vi "8_2.vi"() -> ()   [LabVIEW 2022 SP3]
panel:
  in  "Text.Font:Bold":bool
  in  "Text.Text Colors:Text Color":u32(colorbox)
  out "Text.Selection:Start":u32
  out "Text.Selection:End":u32
  in  "font size":dbl=17.0
  in  "stop":bool
  in  "String":string="Lorem ipsum dolor sit amet, consectetur adipiscing elit, sed do eiusmod tempor incididunt ut labore et dolore magna aliqua. Ut enim ad minim veniam, quis nostrud exercitation ullamco laboris nisi ut aliquip ex ea commodo consequat. Duis aute irure dolor in reprehenderit in voluptate velit esse cillum dolore eu fugiat nulla pariatur. Excepteur sint occaecat cupidatat non proident, sunt in culpa qui officia deserunt mollit anim id est laborum."
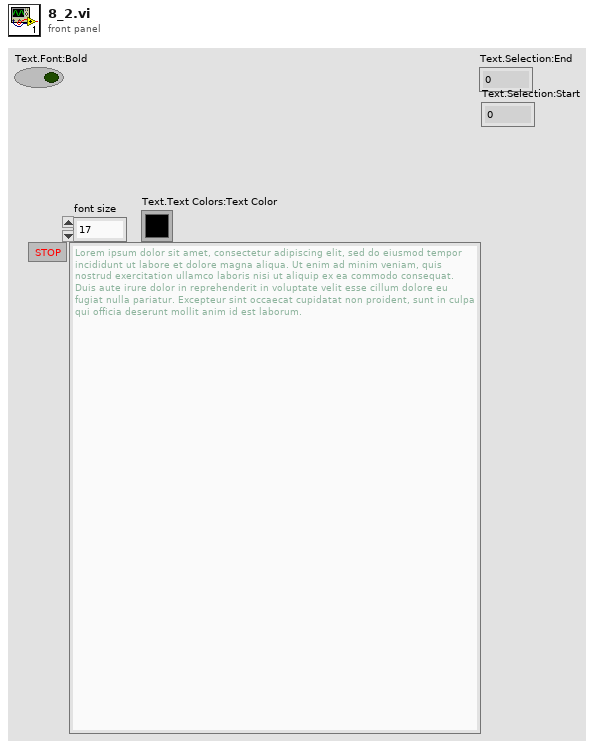
[diagram p1: front panel]
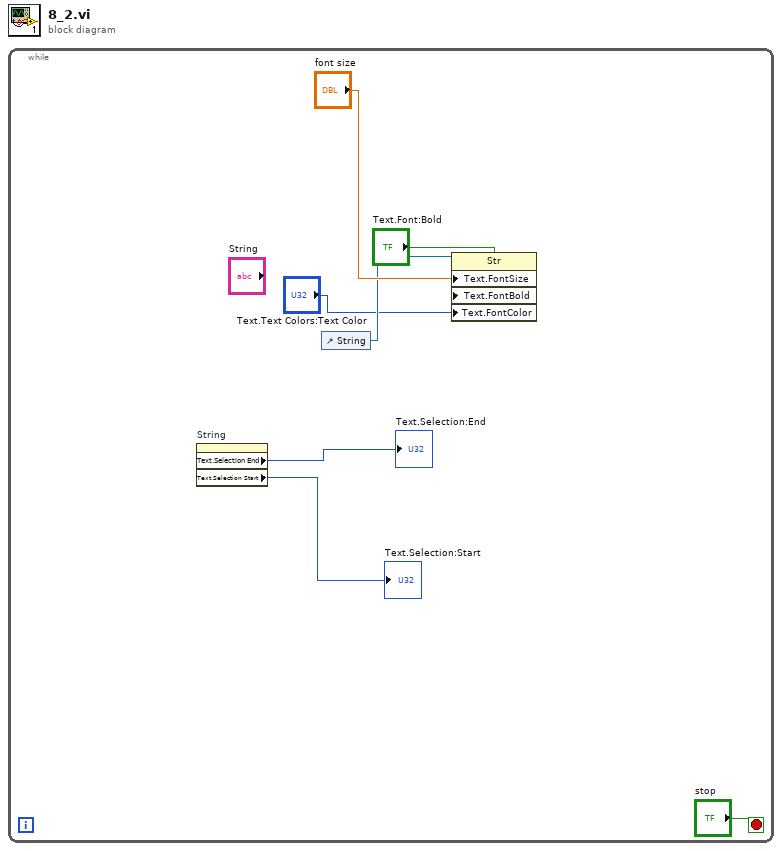
[diagram p0: block diagram]
diagram:
  n1 = while {
    stop <- "stop" stop-if-true
    n2 = property on="String" class="Str"() -> ("Text.Selection End"=→"Text.Selection:End":u32, "Text.Selection Start"=→"Text.Selection:Start":u32)  [unwired: 2 in, 2 out]
    n3 = control-ref of="String"() -> (w5:refnum<vi>)
    n4 = property on="Property Node" class="Str"(reference=w5, "Text.FontSize"="font size", "Text.FontBold"="Text.Font:Bold", "Text.FontColor"="Text.Text Colors:Text Color") -> ()  [unwired: 1 in, 2 out]
  }
